vi "Read ValChange.vi"(8 "error in (no error)":errorcluster, 11 "Tag in":refnum<class "Tag.lvclass">) -> (0 "error out":errorcluster, 2 "ValChange":refnum<user-event>, 3 "Tag out":refnum<class "Tag.lvclass">)   [LabVIEW 2018, in "Tag Engine.lvlib" / "Tag.lvclass"]
uses:
  Tag.lvclass
  Types/ValChange Cluster.ctl
  <vilib>/Utility/Data Type/Type Definitions/Data Type.ctl
  Tag.lvclass/Tag.ctl
  Tag Engine.lvlib
  <vilib>/Utility/Data Type/NI_Data Type.lvlib
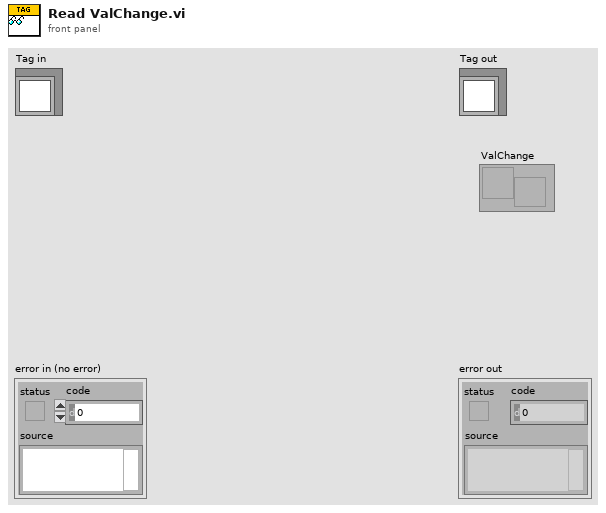
[diagram p1: front panel]
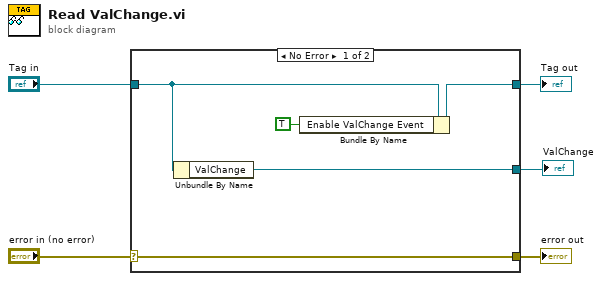
[diagram p0: block diagram]
diagram:
  n1 = case shown="No Error" "error in (no error)" {
    selector: "error in (no error)" -> [w10 w11]
    tunnel: [w10 w11] -> w4
    tunnel: [w9 w12] -> w2
    tunnel: "Tag in" -> [w8 w12]
    tunnel: [w6 _] -> w1
    frame No Error {
      n2 = Unbundle By Name(w8) -> ("ValChange"=w6:refnum<user-event>)
      n3 = Bundle By Name(cluster=w8, "Enable ValChange Event"=TRUE) -> (w9:refnum<class "Tag.lvclass">)
    }
    frame Error {
    }
  }
  "error out" <- w4
  "Tag out" <- w2
  "ValChange" <- w1
